vi "EnumTypeDef.vi"() -> ()   [LabVIEW 2019]
uses:
  States.ctl
panel:
  in  "States 3":T1
  in  "States 2":T1
  in  "States":T1
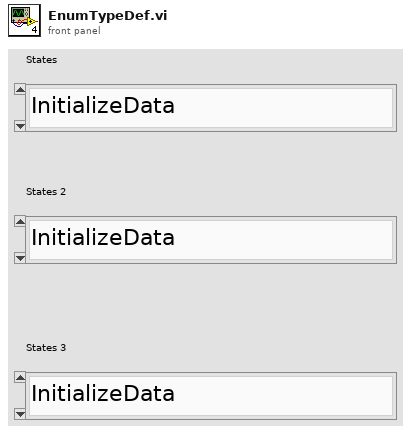
[diagram p1: front panel]
types:
  T1 = typedef "States.ctl" = enum16{"InitializeData", "Initialize", "Process", "Process1", "Process2", "Exit", "MacroExit"}
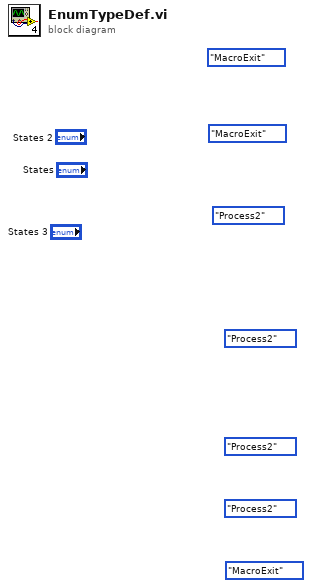
[diagram p0: block diagram]
diagram:
  (unwired) States."MacroExit" ("States")
  (unwired) States."Process2" ("States")
  (unwired) States."Process2" ("States")
  (unwired) States."Process2" ("States")
  (unwired) States."Process2" ("States")
  (unwired) States."MacroExit" ("States")
  (unwired) States."MacroExit" ("States")
